vi "Create Thread.vi"(8 "error in (no error)":errorcluster, 11 "Thread in":refnum<class "Thread.lvclass">) -> (0 "error out":errorcluster, 3 "Thread out":refnum<class "Thread.lvclass">)   [LabVIEW 2016, in "Architecture.lvlib" / "Thread.lvclass"]
uses:
  Thread.lvclass
  Queue/Queue.lvclass
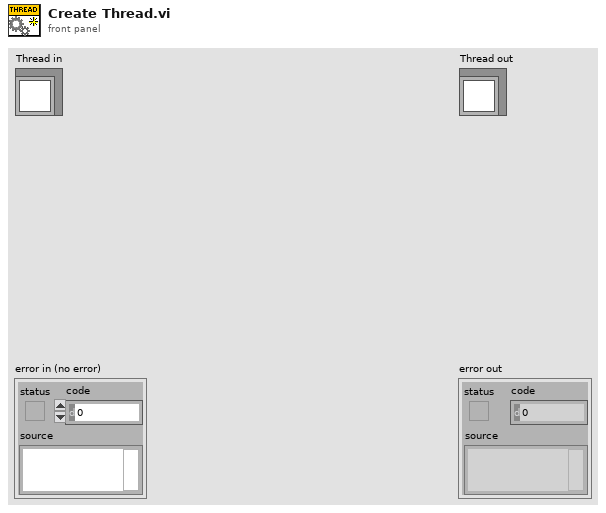
[diagram p1: front panel]
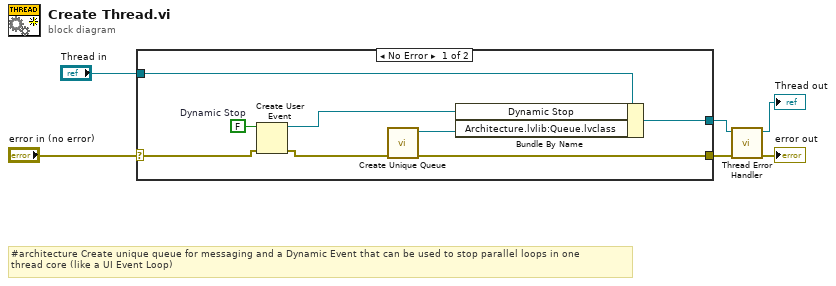
[diagram p0: block diagram]
diagram:
  # "#architecture Create unique queue for messaging and a Dynamic Event that can be used to stop parallel loops in one\nthread core (like a UI Event Loop)"
  n1 = case shown="No Error" "error in (no error)" {
    selector: "error in (no error)" -> [w9 w16]
    tunnel: [w12 w16] -> w4
    tunnel: [w13 w15] -> w1
    tunnel: "Thread in" -> [w14 w15]
    frame No Error {
      w10 = FALSE  # Dynamic Stop
      n2 = Create User Event(user event datatype=w10, error in=w9) -> (user event=w7:refnum<user-event>, error out=w8:errorcluster)
      n3 = call "Create Unique Queue.vi"("error in (no error)"=w8) -> ("error out"=w12:errorcluster, "Queue out"=w11:refnum<class "Queue.lvclass">)  [unwired: 9 in]
      n4 = Bundle By Name(cluster=w14, "Dynamic Stop"=w7, "Architecture.lvlib:Queue.lvclass"=w11) -> (w13:refnum<class "Thread.lvclass">)
    }
    frame Error {
    }
  }
  n5 = call-dynamic "Thread Error Handler.vi"("error in (no error)"=w4, "Thread in"=w1) -> ("error out"=→"error out":errorcluster, "Thread out"=→"Thread out":refnum<class "Thread.lvclass">)  [unwired: 8 in]
